vi "采配水流程与超标留样交互.vi"(11 "参数":T1) -> ()   [LabVIEW 2016, in "PLC.lvlib"]
uses:
  PLC.lvlib
panel:
  out "输出数组":cluster{"参数名":string, "浓度":dbl}[](array[cluster])
  out "数值":i32
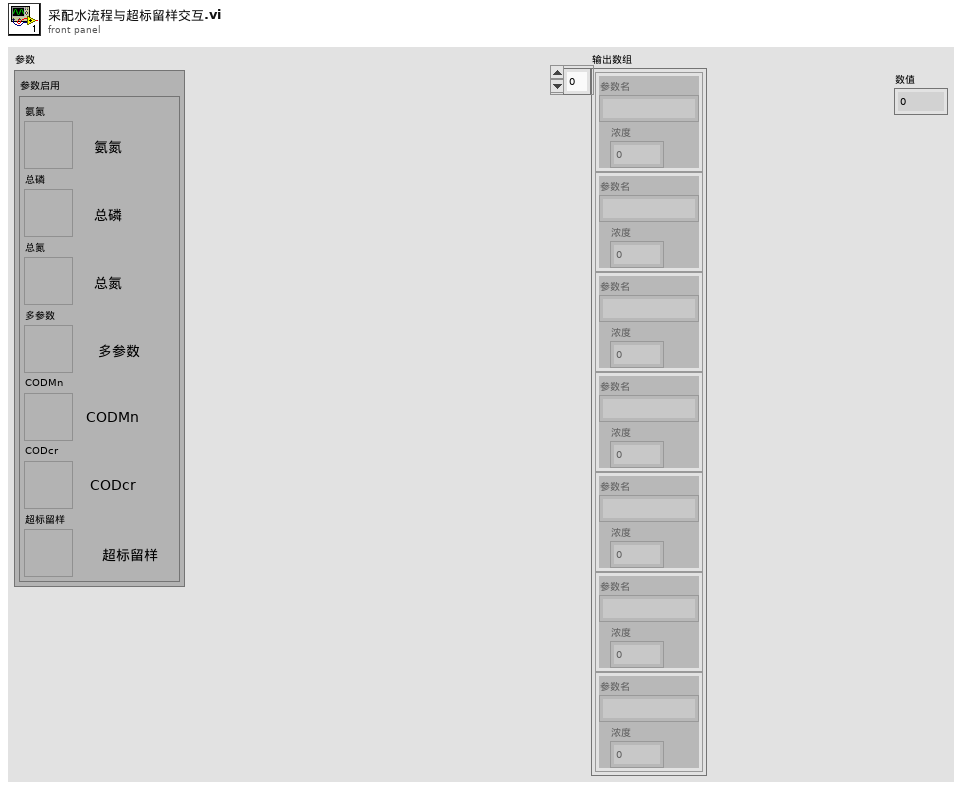
[diagram p1: front panel]
types:
  T1 = cluster{"参数启用":cluster{"氨氮":bool, "总磷":bool, "总氮":bool, "多参数":bool, "CODMn":bool, "CODcr":bool, "超标留样":bool}}
  T2 = cluster{"因子编码":u32, "单位":u16, "标样参考值":sgl, "水样数据时间":timestamp, "水样实测值":sgl, "水样数据标识":string, "标样数据时间":timestamp, "标样实测值":sgl, "标样数据标识":string, "空白数据时间":timestamp, "空白实测值":sgl, "空白数据标识":string, "零点核查数据时间":timestamp, "零点核查实测值":sgl, "零点核查数据标识":string, "跨度核查数据时间":timestamp, "跨度核查实测值":sgl, "跨度核查数据标识":string, "加标回收数据时间":timestamp, "加标回收实测值":sgl, "加标回收数据标识":string, "平行样数据时间":timestamp, "平行样实测值":sgl, "平行样数据标识":string, "F0":sgl, "F1":sgl, "F2":sgl, "F3":sgl, "F4":sgl, "F5":sgl, "F6":sgl, "F7":sgl, "温度":sgl, "湿度":sgl, "X值":sgl, "fidrange":u16}
  T3 = cluster{"因子编码":u32, "单位":u16, "标样参考值":sgl, "水样数据时间":timestamp, "水样实测值":sgl, "水样数据标识":string, "标样数据时间":timestamp, "标样实测值":sgl, "标样数据标识":string, "空白数据时间":timestamp, "空白实测值":sgl, "空白数据标识":string, "零点核查数据时间":timestamp, "零点核查实测值":sgl, "零点核查数据标识":string, "跨度核查数据时间":timestamp, "跨度核查实测值":sgl, "跨度核查数据标识":string, "加标回收数据时间":timestamp, "加标回收实测值":sgl, "加标回收数据标识":string, "平行样数据时间":timestamp, "平行样实测值":sgl, "平行样数据标识":string}
  T4 = cluster{"温度测量值":sgl, "测量值":sgl, "温度偏移修正值":sgl, "信号值":sgl, "数据标识":string}
  T5 = cluster{"温度测量值":sgl, "DO%":sgl, "DOmg/L":sgl, "温度偏移修正值":sgl, "数据标识mg/L":string, "数据标识%":string}
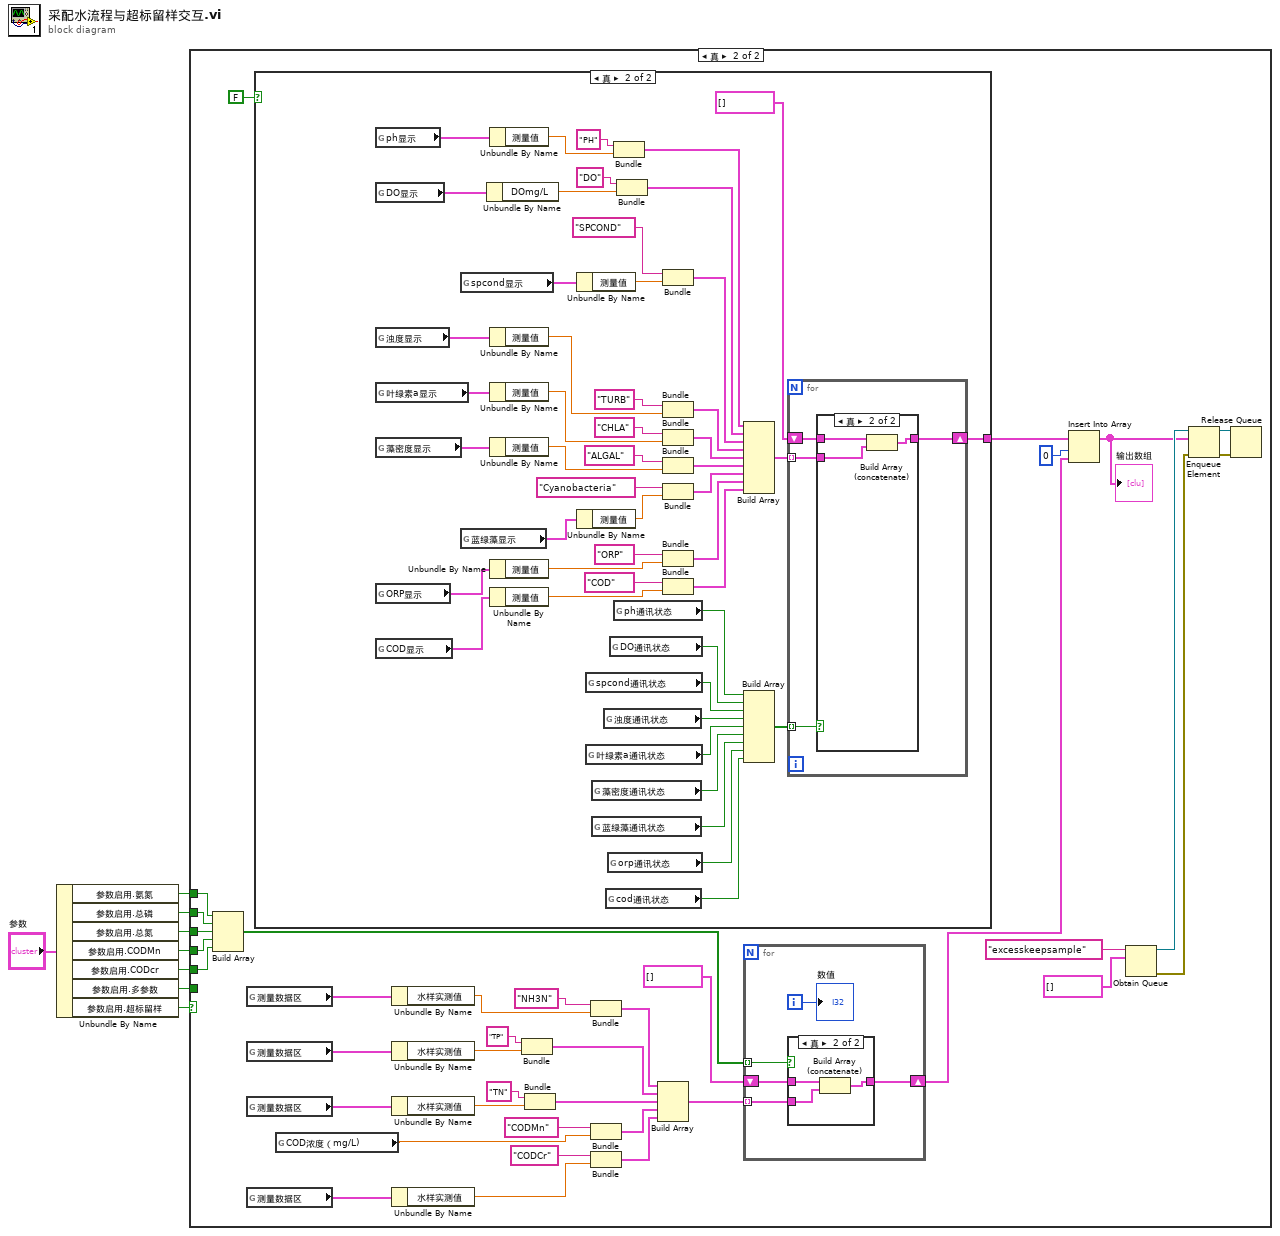
[diagram p0: block diagram]
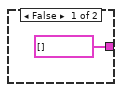
[diagram p4: hidden frame]
diagram:
  n1 = Unbundle By Name("参数") -> ("参数启用.氨氮"=w2:bool, "参数启用.总磷"=w3:bool, "参数启用.总氮"=w4:bool, "参数启用.CODMn"=w5:bool, "参数启用.CODcr"=w6:bool, "参数启用.多参数"=w7:bool, "参数启用.超标留样"=w1:bool)
  n2 = case shown="真" w1 {
    tunnel: w7 -> [_ _]
    tunnel: w6 -> [_ w34]
    tunnel: w5 -> [_ w33]
    tunnel: w4 -> [_ w32]
    tunnel: w3 -> [_ w31]
    tunnel: w2 -> [_ w30]
    frame False {
    }
    frame True {
      n3 = Build Array(w30, w31, w32, w33, w34) -> (w29:bool[])
      n4 = global read "VAR总磷总氮全局变量.vi" "测量数据区"() -> (w41:T2)
      n5 = global read "VAR总磷总氮全局变量.vi" "测量数据区"() -> (w36:T2)
      n6 = global read "VAR总磷总氮全局变量.vi" "测量数据区"() -> (w35:T2)
      n7 = global read "CODcr全局变量.vi" "测量数据区"() -> (w11:T3)
      n8 = case shown="真" FALSE {
        tunnel: [cluster{"参数名":string, "浓度":dbl}[] [] w57] -> w21
        frame False {
        }
        frame True {
          n9 = global read "多参数全局变量.vi" "ph显示"() -> (w89:T4)
          n10 = global read "多参数全局变量.vi" "DO显示"() -> (w105:T5)
          n11 = global read "多参数全局变量.vi" "浊度显示"() -> (w104:T4)
          n12 = global read "多参数全局变量.vi" "叶绿素a显示"() -> (w101:T4)
          n13 = global read "多参数全局变量.vi" "藻密度显示"() -> (w102:T4)
          n14 = global read "多参数全局变量.vi" "ORP显示"() -> (w100:T4)
          n15 = global read "多参数全局变量.vi" "COD显示"() -> (w99:T4)
          n16 = global read "多参数全局变量.vi" "spcond显示"() -> (w81:T4)
          n17 = global read "多参数全局变量.vi" "蓝绿藻显示"() -> (w103:T4)
          n18 = Unbundle By Name(w105) -> ("DOmg/L"=w84:sgl)
          n19 = Unbundle By Name(w89) -> ("测量值"=w88:sgl)
          n20 = Unbundle By Name(w104) -> ("测量值"=w76:sgl)
          n21 = Unbundle By Name(w101) -> ("测量值"=w73:sgl)
          n22 = Unbundle By Name(w102) -> ("测量值"=w71:sgl)
          n23 = Unbundle By Name(w100) -> ("测量值"=w64:sgl)
          n24 = Unbundle By Name(w99) -> ("测量值"=w63:sgl)
          n25 = Unbundle By Name(w81) -> ("测量值"=w80:sgl)
          n26 = Unbundle By Name(w103) -> ("测量值"=w65:sgl)
          n27 = global read "多参数全局变量.vi" "spcond通讯状态"() -> (w96:bool)
          n28 = global read "多参数全局变量.vi" "叶绿素a通讯状态"() -> (w94:bool)
          n29 = global read "多参数全局变量.vi" "藻密度通讯状态"() -> (w93:bool)
          n30 = global read "多参数全局变量.vi" "蓝绿藻通讯状态"() -> (w92:bool)
          n31 = global read "多参数全局变量.vi" "浊度通讯状态"() -> (w95:bool)
          n32 = global read "多参数全局变量.vi" "cod通讯状态"() -> (w90:bool)
          n33 = global read "多参数全局变量.vi" "orp通讯状态"() -> (w91:bool)
          n34 = global read "多参数全局变量.vi" "DO通讯状态"() -> (w97:bool)
          n35 = Bundle("PH", "测量值"=w88) -> (w85:cluster{string, "测量值":sgl})  [unwired: 1 in]
          n36 = global read "多参数全局变量.vi" "ph通讯状态"() -> (w98:bool)
          n37 = Bundle("DO", "DOmg/L"=w84) -> (w82:cluster{string, "DOmg/L":sgl})  [unwired: 1 in]
          n38 = Bundle("SPCOND", "测量值"=w80) -> (w78:cluster{string, "测量值":sgl})  [unwired: 1 in]
          n39 = Bundle("TURB", "测量值"=w76) -> (w75:cluster{string, "测量值":sgl})  [unwired: 1 in]
          n40 = Bundle("CHLA", "测量值"=w73) -> (w70:cluster{string, "测量值":sgl})  [unwired: 1 in]
          n41 = Bundle("ALGAL", "测量值"=w71) -> (w69:cluster{string, "测量值":sgl})  [unwired: 1 in]
          n42 = Bundle("Cyanobacteria", "测量值"=w65) -> (w62:cluster{string, "测量值":sgl})  [unwired: 1 in]
          n43 = Bundle("ORP", "测量值"=w64) -> (w61:cluster{string, "测量值":sgl})  [unwired: 1 in]
          n44 = Bundle("COD", "测量值"=w63) -> (w60:cluster{string, "测量值":sgl})  [unwired: 1 in]
          n45 = Build Array(w85, w82, w78, w75, w70, w69, w62, w61, w60) -> (w59:cluster{string, "测量值":sgl}[])
          n46 = Build Array(w98, w97, w96, w95, w94, w93, w92, w91, w90) -> (w58:bool[])
          n47 = for {
            shift-right: [w108] -> w57
            shift-left: cluster{"参数名":string, "浓度":dbl}[] [] -> [w109]
            tunnel: w59 -> [w107] mode=indexing
            tunnel: w58 -> [w106] mode=indexing
            n48 = case shown="真" w106 {
              tunnel: w109 -> [w110 w113]
              tunnel: [w110 w112] -> w108
              tunnel: w107 -> [_ w111]
              frame False {
              }
              frame True {
                n49 = Build Array (concatenate)(w113, w111) -> (w112:cluster{"参数名":string, "浓度":dbl}[])
              }
            }
          }
        }
      }
      n50 = global read "COD浓度全局变量.vi" "COD浓度（mg/L)"() -> (w9:dbl)
      n51 = Unbundle By Name(w41) -> ("水样实测值"=w43:sgl)
      n52 = Unbundle By Name(w36) -> ("水样实测值"=w39:sgl)
      n53 = Unbundle By Name(w35) -> ("水样实测值"=w38:sgl)
      n54 = Unbundle By Name(w11) -> ("水样实测值"=w44:sgl)
      n55 = Bundle("TP", "水样实测值"=w39) -> (w26:cluster{string, "水样实测值":sgl})  [unwired: 1 in]
      n56 = Bundle("TN", "水样实测值"=w38) -> (w25:cluster{string, "水样实测值":sgl})  [unwired: 1 in]
      n57 = Bundle("NH3N", "水样实测值"=w43) -> (w27:cluster{string, "水样实测值":sgl})  [unwired: 1 in]
      n58 = Bundle("CODMn", "COD浓度（mg/L)"=w9) -> (w24:cluster{string, "COD浓度（mg/L)":dbl})  [unwired: 1 in]
      n59 = Bundle("CODCr", "水样实测值"=w44) -> (w23:cluster{string, "水样实测值":sgl})  [unwired: 1 in]
      n60 = Build Array(w27, w26, w25, w24, w23) -> (w22:cluster{string, "COD浓度（mg/L)":dbl}[])
      n61 = for {
        tunnel: w29 -> [w48] mode=indexing
        shift-right: [w49] -> w19
        shift-left: cluster{"参数名":string, "浓度":dbl}[] [] -> [w51]
        tunnel: w22 -> [w50] mode=indexing
        i -> [w47]
        n62 = case shown="真" w48 {
          tunnel: w51 -> [w52 w55]
          tunnel: w50 -> [_ w54]
          tunnel: [w52 w53] -> w49
          frame False {
          }
          frame True {
            n63 = Build Array (concatenate)(w55, w54) -> (w53:cluster{"参数名":string, "COD浓度（mg/L)":dbl}[])
          }
        }
        "数值" <- w47
      }
      n64 = Insert Into Array(array=w21, index=0 ("索引"), new element=w19) -> (w12:cluster{"参数名":string, "浓度":dbl}[])
      "输出数组" <- w12
      n65 = Obtain Queue(name (unnamed)="excesskeepsample" ("名称（未命名）"), element data type=cluster{"参数名":string, "浓度":dbl}[] []) -> (queue out=w16:refnum<queue>, error out=w15:errorcluster)  [unwired: 3 in, 1 out]
      n66 = Enqueue Element(queue=w16, element=w12, error in (no error)=w15) -> (queue out=w14:refnum<queue>, error out=w13:errorcluster)  [unwired: 1 in, 1 out]
      n67 = Release Queue(queue=w14, error in (no error)=w13) -> ()  [unwired: 1 in, 3 out]
    }
  }
